vi "OP300ZP_Param_ConfZENplusOP100.vi"(8 "errin":errorcluster, 10 "Chaîne":string, 11 "pathin":path) -> (0 "errout":errorcluster, 3 "VISA OUT":T1)   [LabVIEW 2020]
uses:
  <vilib>/Utility/config.llb/Read Key (String).vi
  <vilib>/Utility/config.llb/NI_LVConfig.lvlib
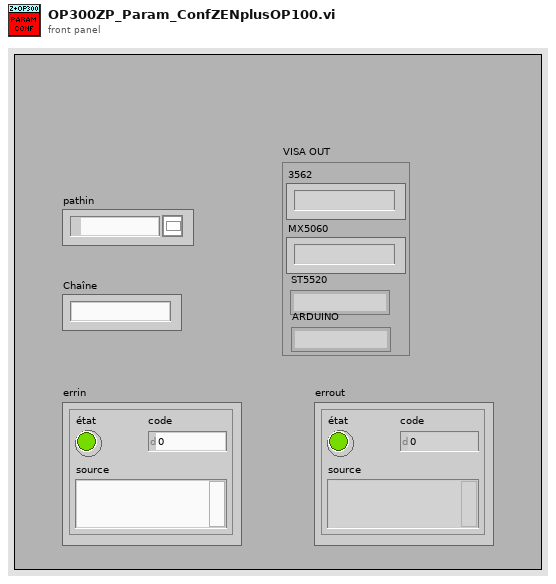
[diagram p1: front panel]
types:
  T1 = cluster{"3562":string, "MX5060":string, "ST5520":string, "ARDUINO":string}
  T2 = typedef "NI_LVConfig.lvlib/Config Data RefNum.ctl" = refnum<k1>
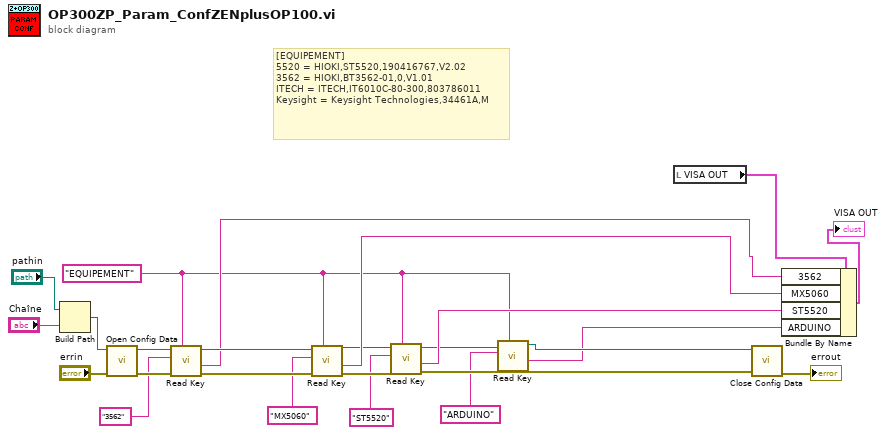
[diagram p0: block diagram]
diagram:
  w2 = "EQUIPEMENT" ("section")
  # "[EQUIPEMENT]\n5520 = HIOKI,ST5520,190416767,V2.02\n3562 = HIOKI,BT3562-01,0,V1.01\nITECH = ITECH,IT6010C-80-300,803786011\nKeysight = Keysight Technologies,34461A,M"
  n1 = Build Path(base path="pathin", name or relative path="Chaîne") -> (appended path=w22:path)
  n2 = call <vilib>:"Open Config Data.vi"("error in (no error)"="errin", "configuration file path"=w22) -> ("error out"=w24:errorcluster, "refnum"=w25:T2)  [unwired: 7 in, 1 out]
  n3 = call-poly <vilib>:"Read Key.vi"("section"=w2, "error in (no error)"=w24, "key"="3562", "refnum"=w25) -> ("error out"=w19:errorcluster, "value"=w13:string, "refnum out"=w21:T2)  [unwired: 4 in, 1 out]
  n4 = call-poly <vilib>:"Read Key.vi"("section"=w2, "error in (no error)"=w19, "key"="MX5060", "refnum"=w21) -> ("error out"=w8:errorcluster, "value"=w12:string, "refnum out"=w7:T2)  [unwired: 4 in, 1 out]
  n5 = call-poly <vilib>:"Read Key.vi"("section"=w2, "error in (no error)"=w8, "key"="ST5520", "refnum"=w7) -> ("error out"=w15:errorcluster, "value"=w11:string, "refnum out"=w5:T2)  [unwired: 4 in, 1 out]
  n6 = call-poly <vilib>:"Read Key.vi"("section"=w2, "key"="ARDUINO", "refnum"=w5) -> ("value"=w1:string, "refnum out"=w4:T2)  [unwired: 5 in, 2 out]
  n7 = local read "VISA OUT"() -> (w14:T1)
  n8 = call <vilib>:"Close Config Data.vi"("error in (no error)"=w15, "refnum"=w4) -> ("error out"=→"errout":errorcluster)  [unwired: 8 in, 1 out]
  n9 = Bundle By Name(cluster=w14, "3562"=w13, "MX5060"=w12, "ST5520"=w11, "ARDUINO"=w1) -> (→"VISA OUT":T1)
